vi "ArmSetXZDemand.vi"(8 "error in (no error)":errorcluster, 9 "SetZ":dbl, 11 "SetX":dbl) -> (0 "error out":errorcluster, 2 "Extend":dbl, 3 "Lift":dbl)   [LabVIEW 2020]
doc: "Set XYZ demand for X,Y,Z arm globals and for ArmXYZToR-L-E, and set those outputs to ArmSetDemands\n\nInputs:\n--SetX--Double\n--SetY--Double\n--SetZ--Double"
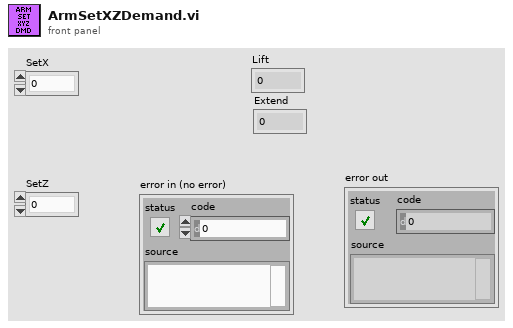
[diagram p1: front panel]
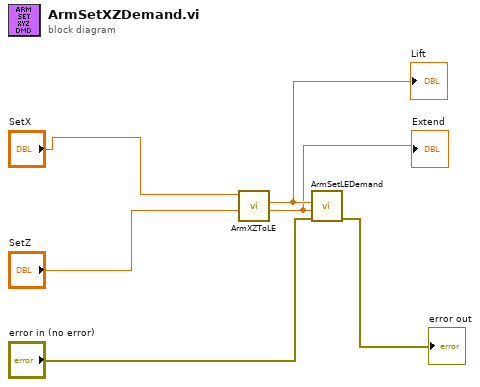
[diagram p0: block diagram]
diagram:
  n1 = call "ArmXZToLE.vi"("Z"="SetZ", "X"="SetX") -> ("Extend"=w3:dbl, "Lift"=w4:dbl)  [unwired: 8 in]
  "Lift" <- w4
  "Extend" <- w3
  n2 = call "ArmSetLEDemand.vi"("error in (no error)"="error in (no error)", "SetExtendPositonDemand(in)"=w3, "SetLIftPostionDemand(d)"=w4) -> ("error out"=→"error out":errorcluster)  [unwired: 8 in]
